vi "LVH5Rcreate (DSet).vi"(6 "error in (no error)":errorcluster, 7 "HDF5 Space Ref":T1, 8 "Name":string, 9 "HDF5 Loc Ref":T1) -> (0 "error out":errorcluster, 2 "HDF5 Dataset Region Reference":T2, 3 "HDF5 Loc Ref out":T1)   [LabVIEW 2017]
doc: "Creates a reference."
uses:
  <vilib>/UPVI/lvhdf5/library.llb/HDF5 Ref.ctl
  <vilib>/UPVI/lvhdf5/reference.llb/H5R Dataset Region Ref.ctl
  <vilib>/UPVI/lvhdf5/reference.llb/H5R_type_t.ctl
  <vilib>/UPVI/lvhdf5/h5helper.dll
panel:
  # "LVHDF5 Toolkit\nCopyright (c) 2005-2013 by Jason D. Sommerville\nCopyright (c) 2014 by UPVI, LLC.\n\nThis use and distribution of this file is governed by the terms found in \nLICENSE.txt distributed with this toolkit and installed at\n <user.lib>\\_lvhdf5\\LICENSE.txt"
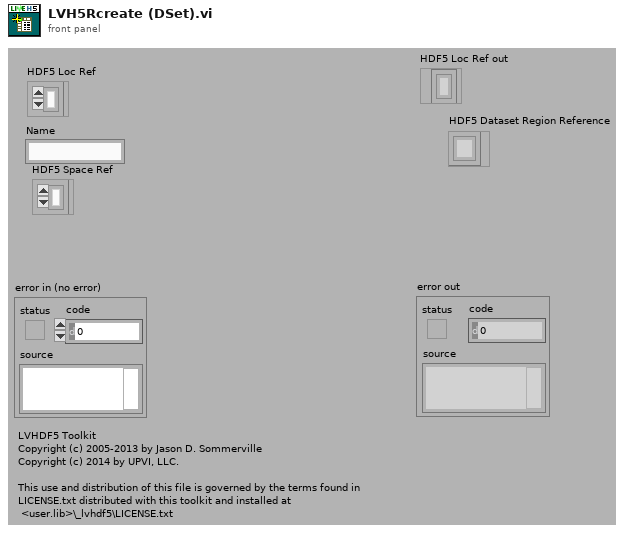
[diagram p1: front panel]
types:
  T1 = typedef "HDF5 Ref.ctl" = refnum<k1>
  T2 = typedef "H5R Dataset Region Ref.ctl" = refnum<k1>
  T3 = typedef "H5R_type_t.ctl" = i32
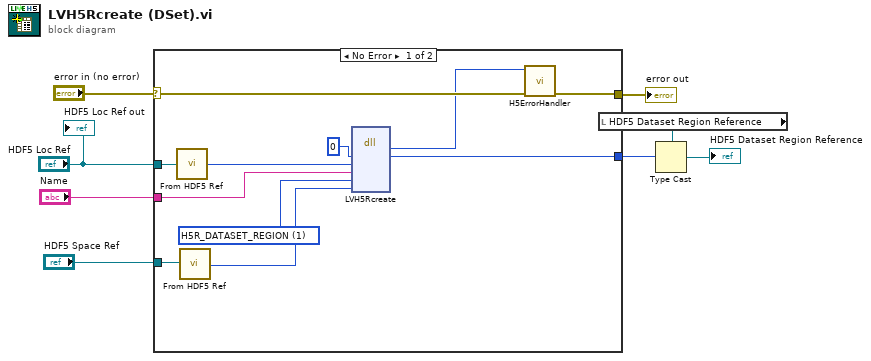
[diagram p0: block diagram]
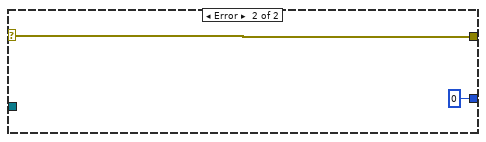
[diagram p2: hidden frame]
diagram:
  n1 = case shown="No Error" "error in (no error)" {
    selector: "error in (no error)" -> [w19 w21]
    tunnel: [w18 w21] -> w7
    tunnel: "HDF5 Loc Ref" -> [w16 _]
    tunnel: "Name" -> [w13 _]
    tunnel: [w11 0 ("pHandle")] -> w4
    tunnel: "HDF5 Space Ref" -> [w10 _]
    frame No Error {
      w14 = T3 1 items=["H5R_BADTYPE"=-1, "H5R_OBJECT"=0, "H5R_DATASET_REGION"=1, "H5R_INTERNAL"=2] ("Reference Type")
      n2 = call <vilib>:"From HDF5 Ref.vi"("HDF5 Ref"=w16) -> ("I32"=w15:i32)
      n3 = call <vilib>:"From HDF5 Ref.vi"("HDF5 Ref"=w10) -> ("I32"=w9:i32)
      n4 = dll-call lib="C:/Program Files/National Instruments/LabVIEW 2017/vi.lib/UPVI/lvhdf5/h5helper.dll" fn="LVH5Rcreate"("pHandle"=0, "loc_id"=w15, "name"=w13, "ref_type"=w14, "space_id"=w9) -> (w17:i32, "pHandle"=w11:i32)  [unwired: 7 in, 2 out]
      n5 = call <vilib>:"H5ErrorHandler.vi"("error in (no error)"=w19, "herr_t"=w17) -> ("error out"=w18:errorcluster)  [unwired: 3 in, 4 out]
    }
    frame Error {
    }
  }
  "error out" <- w7
  n6 = local read "HDF5 Dataset Region Reference"() -> (w5:T2)
  n7 = Type Cast(type=w5, x=w4) -> (*(type *) &x=→"HDF5 Dataset Region Reference":T2)
  "HDF5 Loc Ref out" <- "HDF5 Loc Ref"
